vi "Button RefNum to Num.vi"(8 "error in (no error)":errorcluster, 11 "Button Reference":refnum<vi>) -> (0 "error out":errorcluster, 2 "Number on Button":dbl)   [LabVIEW 2014]
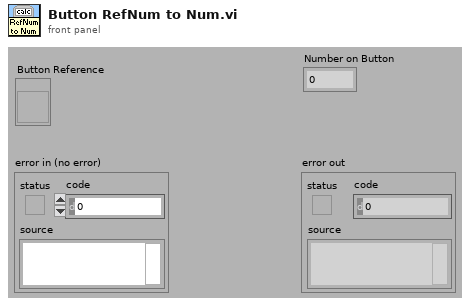
[diagram p1: front panel]
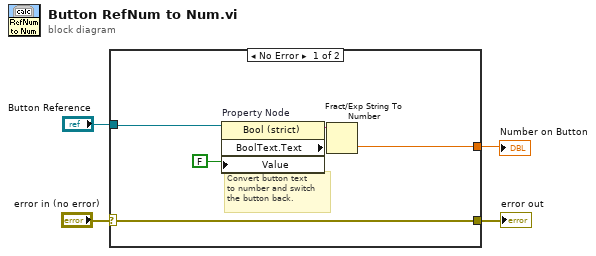
[diagram p0: block diagram]
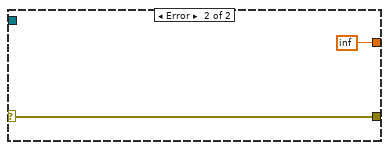
[diagram p2: hidden frame]
diagram:
  n1 = case shown="No Error" "error in (no error)" {
    selector: "error in (no error)" -> [w7 w11]
    tunnel: [w9 inf] -> w4
    tunnel: [w7 w11] -> w2
    tunnel: "Button Reference" -> [w6 _]
    frame No Error {
      # "Convert button text\nto number and switch the button back."
      n2 = property on="Property Node" class="Bool (strict)"(reference=w6, "Value"=FALSE) -> ("BoolText.Text"=w8:string)  [unwired: 1 in, 2 out]
      n3 = Fract/Exp String To Number(string=w8) -> (number=w9:dbl)  [unwired: 3 in, 1 out]
    }
    frame Error {
    }
  }
  "Number on Button" <- w4
  "error out" <- w2
